vi "快捷键.vi"() -> ()   [LabVIEW 2010]
panel:
  in  "停止":bool
  in  "字符串":string="LabVIEW2010"
  out "仪表":dbl(knob)=5.000026307457805 scale=0.0..10.0
  in  "数值":dbl=5.0 step=0.2
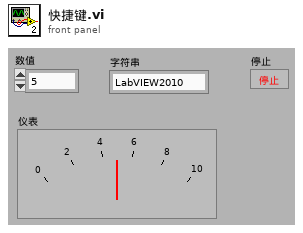
[diagram p1: front panel]
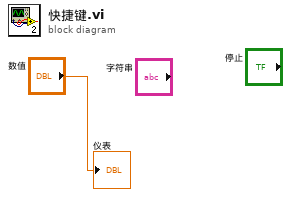
[diagram p0: block diagram]
diagram:
  "仪表" <- "数值"
